vi "Fetch Histogram.vi"(8 "error in (no error)":errorcluster, 10 "Timeout (10000 ms)":u32=10000, 11 "VISA resource name":refnum<visa-resource-name>) -> (0 "error out":errorcluster, 1 "Data":dbl[](array[numeric]), 2 "Number of Measurement":dbl, 3 "VISA resource name out":refnum<visa-resource-name>, 4 "Upper Range Value":dbl format="%#_12g", 5 "Lower Range Value":dbl format="%#_16g")   [LabVIEW 2021, in "Agilent 532XX Series.lvlib"]
doc: "Queries and retrieves histogram measurement.\n\n<B>Note:</B> This VI does not check the instrument status. Typically, you call this VI only in a sequence of calls to other low-level instrument driver VIs. The sequence performs one operation. You use the low-level VIs to optimize one or more aspects of interaction with the instrument."
uses:
  <instrlib>/Agilent 532XX Series/Agilent 532XX Series.lvlib
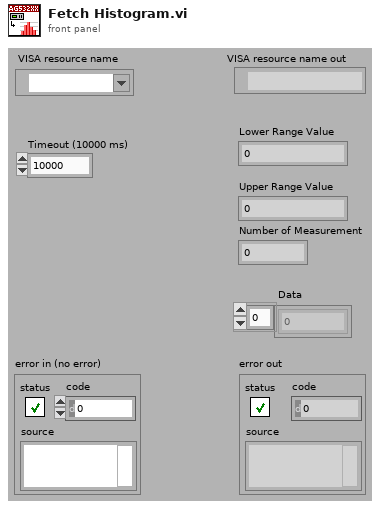
[diagram p1: front panel]
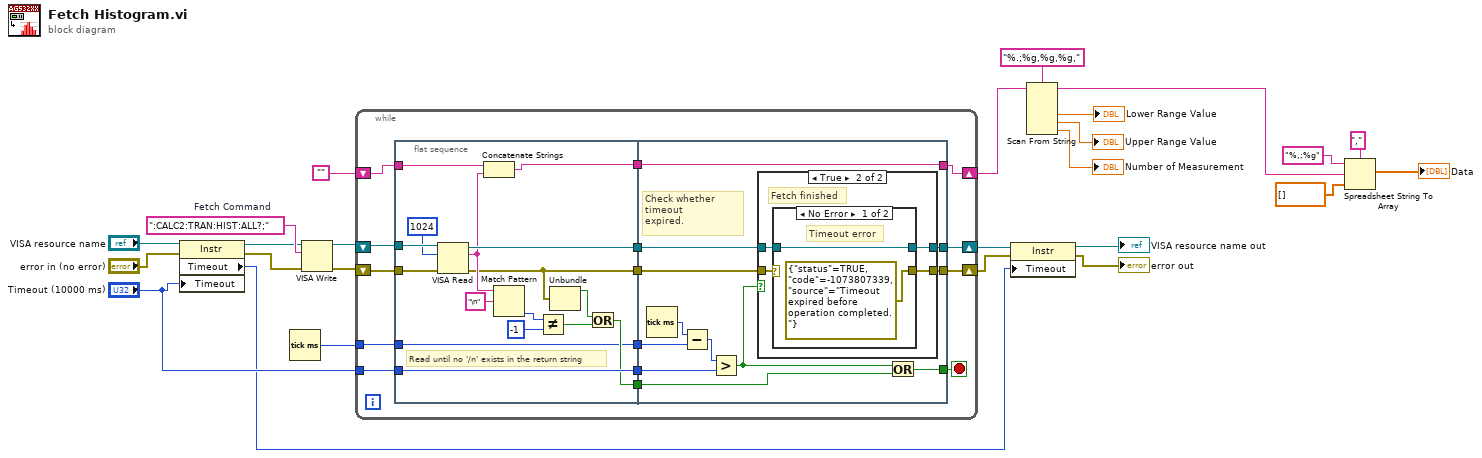
[diagram p0: block diagram]
diagram:
  w23 = ":CALC2:TRAN:HIST:ALL?;"  # Fetch Command
  n1 = property on="Property Node" class="Instr"(reference="VISA resource name", error in="error in (no error)", "Timeout"="Timeout (10000 ms)") -> (reference out=w19:refnum<visa-resource-name>, error out=w20:errorcluster, "Timeout"=w15:u32)
  n2 = Tick Count (ms)() -> (millisecond timer value=w17:u32)
  n3 = VISA Write(VISA resource name=w19, write buffer=w23, error in (no error)=w20) -> (VISA resource name out=w8:refnum<visa-resource-name>, error out=w7:errorcluster)  [unwired: 1 out]
  n4 = while {
    shift-right: [w36] -> w4
    shift-left: "" ("Empty String Constant") -> [w37]
    tunnel: w17 -> [w30]
    tunnel: "Timeout (10000 ms)" -> [w29]
    shift-right: [w39] -> w14
    shift-left: w8 -> [w38]
    shift-right: [w35] -> w13
    shift-left: w7 -> [w40]
    stop <- w26 stop-if-true
    n5 = flat-sequence {
      tunnel: w40 -> [w56]
      tunnel: w38 -> [w54]
      tunnel: w37 -> [w52]
      tunnel: [w55] -> w34
      tunnel: [w51] -> w33
      tunnel: [w46] -> w32
      tunnel: [w41] -> w31
      tunnel: w30 -> [w41]
      tunnel: w29 -> [w44]
      tunnel: [w44] -> w28
      tunnel: [w42] -> w27
      tunnel: [w63] -> w35
      tunnel: [w68] -> w36
      tunnel: [w60] -> w39
      tunnel: w34 -> [w61]
      tunnel: w33 -> [w68]
      tunnel: w32 -> [w62]
      tunnel: w31 -> [w66]
      tunnel: w28 -> [w64]
      tunnel: w27 -> [w59]
      tunnel: [w57] -> w26
      frame #0 {
        # "Read until no '/n' exists in the return string"
        n6 = VISA Read(VISA resource name=w54, byte count=u32 1024, error in (no error)=w56) -> (VISA resource name out=w55:refnum<visa-resource-name>, read buffer=w50:string, error out=w46:errorcluster)  [unwired: 1 out]
        n7 = Concatenate Strings(w52, w50) -> (w51:string)
        n8 = Match Pattern(string=w50, regular expression="\n") -> (offset past match=w49:i32)  [unwired: 4 out]
        n9 = Not Equal?(x=w49, y=-1) -> (x != y?=w45:bool)
        n10 = Unbundle(w46) -> ("status"=w43:bool)  [unwired: 2 out]
        n11 = Or(x=w43, y=w45) -> (x .or. y?=w42:bool)
      }
      frame #1 {
        # "Check whether timeout\nexpired."
        n12 = Tick Count (ms)() -> (millisecond timer value=w67:u32)
        n13 = Subtract(x=w67, y=w66) -> (x-y=w65:u32)
        n14 = Greater?(x=w65, y=w64) -> (0:w58:bool)
        n15 = case shown="True" w58 {
          tunnel: [w70 w74] -> w63
          tunnel: w62 -> [w70 w71]
          tunnel: w61 -> [w69 w73]
          tunnel: [w69 w72] -> w60
          frame False {
            # "continue fetch"
          }
          frame True {
            # "Fetch finished"
            n16 = case shown="No Error" w71 {
              selector: w71 -> [_ w77]
              tunnel: [errorcluster {"status"=TRUE, "code"=-1073807339, "source"="Timeout expired before operation completed."} ("error out") w77] -> w74
              tunnel: w73 -> [w75 w78]
              tunnel: [w75 w78] -> w72
              frame No Error {
                # "Timeout error"
              }
              frame Error {
              }
            }
          }
        }
        n17 = Or(x=w58, y=w59) -> (x .or. y?=w57:bool)
      }
    }
  }
  n18 = property on="Property Node" class="Instr"(reference=w14, error in=w13, "Timeout"=w15) -> (reference out=→"VISA resource name out":refnum<visa-resource-name>, error out=→"error out":errorcluster)
  n19 = Scan From String(format string="%.;%g,%g,%g,", input string=w4) -> (remaining string=w3:string, output 1=→"Lower Range Value":dbl, output 2=→"Upper Range Value":dbl, output 3=→"Number of Measurement":dbl)  [unwired: 2 in, 5 out]
  n20 = Spreadsheet String To Array(delimiter (Tab)=",", format string="%,;%g", spreadsheet string=w3, array type (2D Dbl)=dbl[] [] ("Results")) -> (array=→"Data":dbl[])
